vi "q3.vi"() -> ()   [LabVIEW 2015]
panel:
  out "Carrier Wave":dbl[](graph)=[1.0, -1.0, 1.0, -1.0, 1.0, -1.0, 1.0, -1.0, 1.0, -1.0, 1.0, -1.0, 1.0, -1.0, 1.0, -1.0, 1.0, -1.0, 1.0, -1.0, 1.0, -1.0, 1.0, -1.0, 1.0, -1.0, 1.0, -1.0, 1.0, -1.0, 1.0, -1.0, 1.0, -1.0, 1.0, -1.0, 1.0, -1.0, 1.0, -1.0, 1.0, -1.0, 1.0, -1.0, 1.0, -1.0, 1.0, -1.0, 1.0, -1.0, 1.0, -1.0, 1.0, -1.0, 1.0, -1.0, 1.0, -1.0, 1.0, -1.0, 1.0, -1.0, 1.0, -1.0, 1.0, -1.0, 1.0, -1.0, 1.0, -1.0, 1.0, -1.0, 1.0, -1.0, 1.0, -1.0, 1.0, -1.0, 1.0, -1.0]
  out "Integrated Wave":dbl[](graph)=[0.0, 0.0029389262614623658, 0.0076942088429381335, 0.0124494914244139, 0.015388417685876267, 0.015388417685876267, 0.0124494914244139, 0.007694208842938133, 0.0029389262614623645, -2.168404344971009e-18, -3.393051144118362e-18, 0.0029389262614623645, 0.0076942088429381335, 0.012449491424413902, 0.015388417685876269, 0.01538841768587627, 0.012449491424413907, 0.007694208842938137, 0.002938926261462368, 4.336808689942018e-19, -2.0156127293005046e-18, 0.0029389262614623614, 0.007694208842938132, 0.012449491424413898, 0.015388417685876258, 0.015388417685876262, 0.0124494914244139, 0.007694208842938133, 0.0029389262614623636, 9.540979117872439e-18, 5.86703872043038e-18, 0.0029389262614623684, 0.007694208842938135, 0.012449491424413903, 0.015388417685876258, 0.015388417685876262, 0.0124494914244139, 0.0076942088429381335, 0.0029389262614623645, 9.540979117872439e-18, 4.642391921283026e-18, 0.0029389262614623805, 0.007694208842938147, 0.012449491424413917, 0.015388417685876274, 0.015388417685876279, 0.012449491424413903, 0.007694208842938137, 0.0029389262614623723, 1.6046192152785466e-17, 9.9229581570487e-18, 0.0029389262614623853, 0.007694208842938152, 0.012449491424413917, 0.015388417685876288, 0.015388417685876312, 0.012449491424413952, 0.007694208842938181, 0.0029389262614624217, 6.505213034913027e-17, 5.770424955424615e-17, 0.0029389262614624317, 0.007694208842938198, 0.012449491424413962, 0.015388417685876335, 0.015388417685876324, 0.012449491424413966, 0.007694208842938195, 0.0029389262614624356, 7.762887554996212e-17, 6.905634795593064e-17, 0.0029389262614624417, 0.007694208842938206, 0.012449491424413971, 0.015388417685876343, 0.015388417685876371, 0.012449491424414013, 0.007694208842938242, 0.0029389262614624824, 1.235990476633475e-16]
  out "Modulated Graph":dbl[](graph)=[1.0, -0.9325743402914628, 0.5678681150392391, -0.006347052184169686, -0.355051607843563, 0.3550516078435662, 0.006347052184168277, -0.5678681150392366, 0.9325743402914636, -1.0, 1.0, -0.9325743402914625, 0.5678681150392402, -0.006347052184165582, -0.3550516078435685, 0.35505160784356504, 0.006347052184169501, -0.5678681150392377, 0.932574340291464, -1.0, 1.0, -0.9325743402914629, 0.5678681150392353, -0.006347052184159701, -0.3550516078435607, 0.35505160784356393, 0.006347052184163621, -0.5678681150392328, 0.9325743402914594, -1.0, 1.0, -0.9325743402914608, 0.5678681150392422, -0.00634705218416803, -0.3550516078435662, 0.3550516078435561, 0.006347052184171951, -0.5678681150392397, 0.9325743402914624, -1.0, 1.0, -0.9325743402914638, 0.5678681150392373, -0.0063470521841621505, -0.3550516078435717, 0.3550516078435616, 0.00634705218416607, -0.5678681150392348, 0.9325743402914602, -1.0, 1.0, -0.9325743402914617, 0.5678681150392324, -0.00634705218415627, -0.3550516078435772, 0.35505160784356715, 0.006347052184131769, -0.5678681150392534, 0.9325743402914581, -1.0, 1.0, -0.9325743402914596, 0.5678681150392276, -0.006347052184150389, -0.35505160784355616, 0.35505160784357265, 0.006347052184154309, -0.5678681150392252, 0.932574340291456, -1.0, 1.0, -0.9325743402914575, 0.5678681150392462, -0.006347052184144508, -0.3550516078435616, 0.35505160784355155, 0.006347052184148428, -0.5678681150392437, 0.9325743402914539, -1.0]
  in  "Fc":dbl=100.0
  in  "deF":dbl=20.0
  out "Modulating wave":dbl[](graph)=[0.0, 0.5877852522924731, 0.9510565162951535, 0.9510565162951535, 0.5877852522924732, 1.2246467991473532e-16, -0.5877852522924734, -0.9510565162951535, -0.9510565162951536, -0.5877852522924734, -2.4492935982947064e-16, 0.5877852522924736, 0.9510565162951538, 0.9510565162951536, 0.5877852522924734, 3.6739403974420594e-16, -0.5877852522924728, -0.951056516295154, -0.9510565162951538, -0.5877852522924735, -4.898587196589413e-16, 0.5877852522924727, 0.951056516295154, 0.9510565162951532, 0.5877852522924721, 6.123233995736766e-16, -0.5877852522924726, -0.9510565162951534, -0.9510565162951538, -0.5877852522924708, -7.347880794884119e-16, 0.5877852522924725, 0.9510565162951533, 0.9510565162951539, 0.5877852522924709, 8.572527594031472e-16, -0.5877852522924724, -0.9510565162951533, -0.9510565162951539, -0.587785252292471, -9.797174393178826e-16, 0.5877852522924751, 0.9510565162951533, 0.9510565162951539, 0.5877852522924711, 1.102182119232618e-15, -0.5877852522924751, -0.9510565162951532, -0.9510565162951529, -0.5877852522924712, -1.2246467991473533e-15, 0.587785252292475, 0.9510565162951532, 0.9510565162951529, 0.5877852522924742, 4.899825157862589e-15, -0.587785252292472, -0.9510565162951542, -0.9510565162951519, -0.5877852522924714, -1.4695761589768238e-15, 0.5877852522924748, 0.9510565162951531, 0.951056516295153, 0.5877852522924744, -1.9606728399089416e-15, -0.5877852522924718, -0.9510565162951542, -0.9510565162951519, -0.5877852522924716, -1.7145055188062944e-15, 0.5877852522924746, 0.951056516295153, 0.951056516295153, 0.5877852522924746, 5.3896838775215305e-15, -0.5877852522924716, -0.9510565162951541, -0.951056516295152, -0.5877852522924718]
  out "Numeric":dbl=1.235990476633475e-16
  in  "Amplitude":dbl=1.0
  in  "Fs":dbl=200.0
  in  "phase":dbl
  in  "Frequency":dbl=20.0
  out "Numeric 3":dbl=79.0
  in  "No of Iteration":i32=80
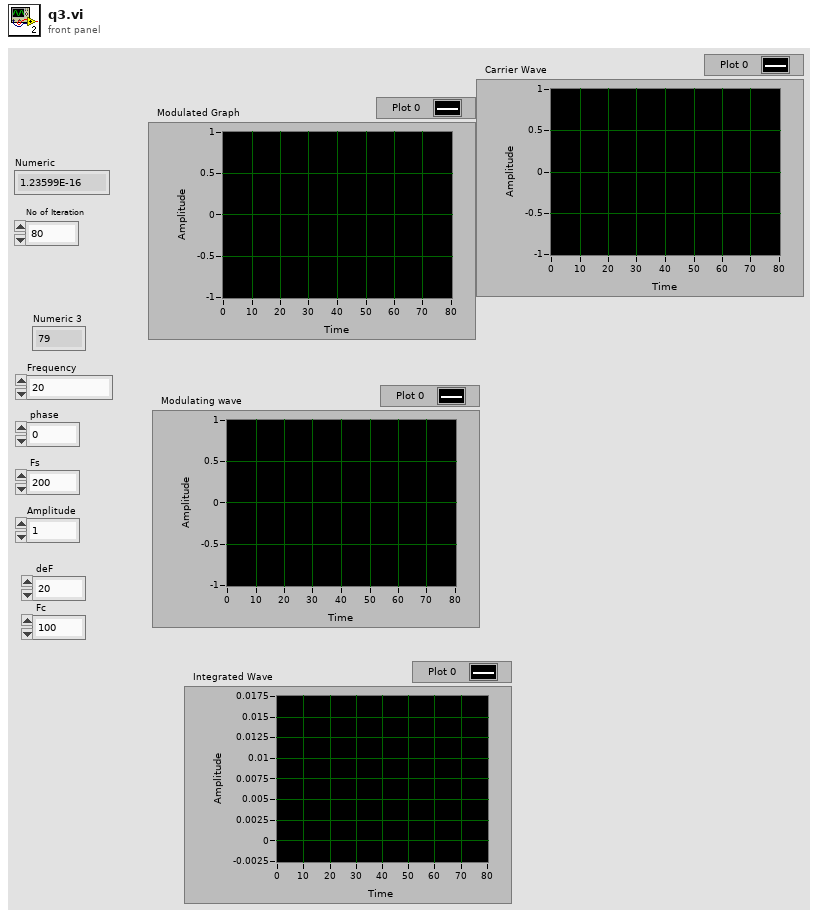
[diagram p1: front panel]
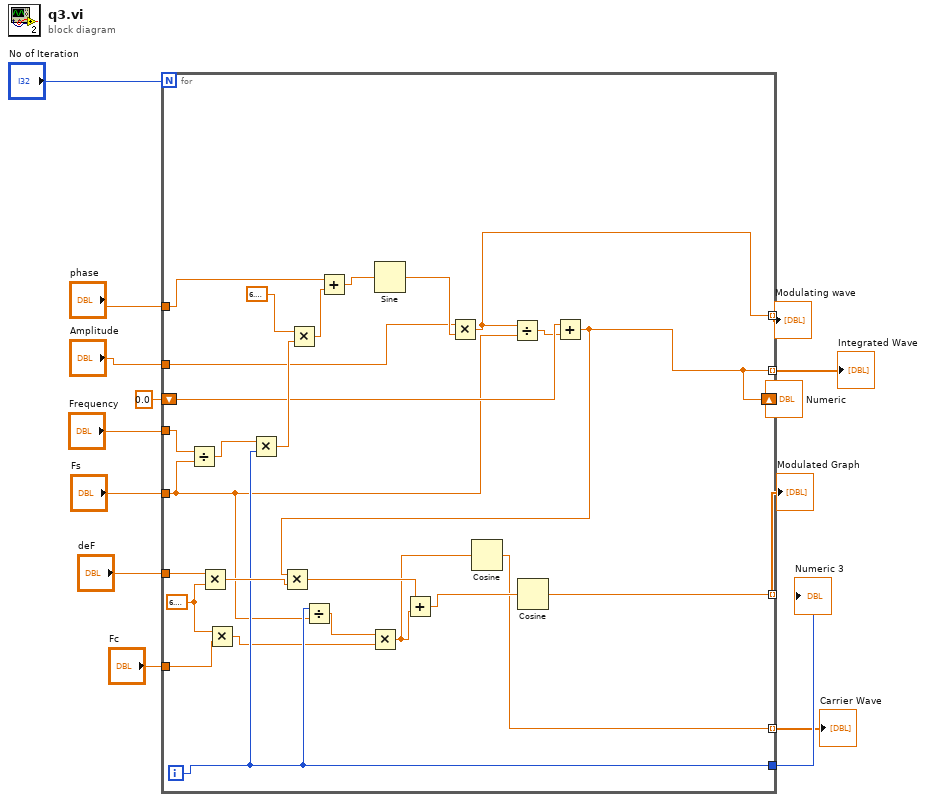
[diagram p0: block diagram]
diagram:
  n1 = for {
    N: "No of Iteration" -> [_]
    tunnel: [w24] -> w14
    tunnel: "Frequency" -> [w39]
    tunnel: "Fs" -> [w23]
    tunnel: "Amplitude" -> [w35]
    tunnel: "phase" -> [w34]
    shift-right: [w18] -> w8
    shift-left: 0.0 -> [w32]
    tunnel: [w29] -> w7 mode=indexing
    tunnel: "deF" -> [w28]
    tunnel: "Fc" -> [w25]
    tunnel: [w19] -> w3 mode=indexing
    tunnel: [w18] -> w2 mode=indexing
    tunnel: [w15] -> w1 mode=indexing
    i -> [w24]
    w26 = 6.283185307179586
    n2 = Divide(x=w39, y=w23) -> (x/y=w33:dbl)
    n3 = Multiply(x=w28, y=w26) -> (x*y=w27:dbl)
    n4 = Multiply(x=w26, y=w25) -> (x*y=w22:dbl)
    n5 = Multiply(x=w33, y=w24) -> (x*y=w37:dbl)
    n6 = Multiply(x=6.283185307179586, y=w37) -> (x*y=w38:dbl)
    n7 = Divide(x=w24, y=w23) -> (x/y=w21:dbl)
    n8 = Add(x=w34, y=w38) -> (x+y=w40:dbl)
    n9 = Multiply(x=w21, y=w22) -> (x*y=w16:dbl)
    n10 = Sine(x=w40) -> (sin(x)=w36:dbl)
    n11 = Multiply(x=w35, y=w36) -> (x*y=w29:dbl)
    n12 = Cosine(x=w16) -> (cos(x)=w15:dbl)
    n13 = Divide(x=w29, y=w23) -> (x/y=w30:dbl)
    n14 = Add(x=w32, y=w30) -> (x+y=w18:dbl)
    n15 = Multiply(x=w18, y=w27) -> (x*y=w17:dbl)
    n16 = Add(x=w17, y=w16) -> (x+y=w20:dbl)
    n17 = Cosine(x=w20) -> (cos(x)=w19:dbl)
  }
  "Numeric 3" <- w14
  "Numeric" <- w8
  "Modulating wave" <- w7
  "Modulated Graph" <- w3
  "Integrated Wave" <- w2
  "Carrier Wave" <- w1
